vi "Derivative x(t).vi"(6 "method":u16(ring) items=["2nd Order Central", "4th Order Central", "Forward", "Backward"], 8 "dt":dbl=1.0 format="%0.2f", 9 "Final Condition":dbl[](array[numeric])=[0.0] format="%#_6f", 10 "Initial Condition":dbl[](array[numeric])=[0.0] format="%#_6f", 11 "X":dbl[](array[numeric])) -> (0 "error":i32, 3 "dX/dt":dbl[](array[numeric]))   [LabVIEW 2010, in "NI_AALPro.lvlib"]
doc: "Performs a discrete differentiation of the sampled signal <B>X</B>."
uses:
  NI_AALPro.lvlib
  lvanlys.dll
panel:
  # "dx(t)/dt"
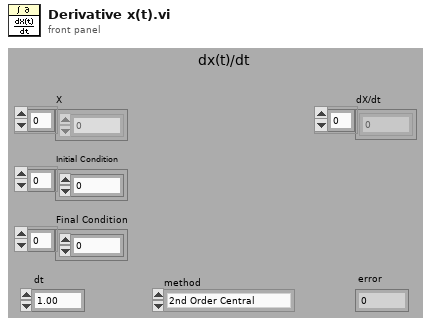
[diagram p1: front panel]
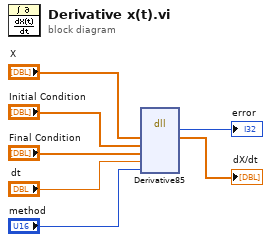
[diagram p0: block diagram]
diagram:
  n1 = dll-call lib="C:/Program Files/National Instruments/LabVIEW 2010/resource/lvanlys.*" fn="Derivative85"("X"="X", "initial condition"="Initial Condition", "final condition"="Final Condition", "dt"="dt", "diffType"="method") -> ("return type"=→"error":i32, "X"=→"dX/dt":dbl[])  [unwired: 6 in, 3 out]
